vi "GetStringBetweenMatches.vi"(9 "postTarget":string, 10 "preTarget":string, 11 "stringIn":string) -> (0 "remainingString":string, 3 "target":string)   [LabVIEW 2020]
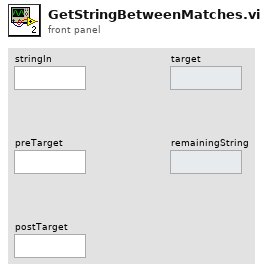
[diagram p1: front panel]
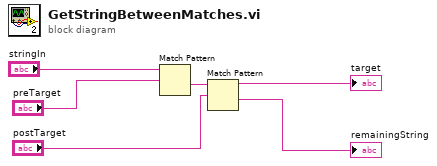
[diagram p0: block diagram]
diagram:
  n1 = Match Pattern(string="stringIn", regular expression="preTarget") -> (after substring=w3:string)  [unwired: 1 in, 3 out]
  n2 = Match Pattern(string=w3, regular expression="postTarget") -> (before substring=→"target":string, after substring=→"remainingString":string)  [unwired: 1 in, 2 out]
